vi "solar Delete Target COSMOS Files.vi"(7 "Config Path":path, 8 "error in (no error)":errorcluster, 10 "Target":string, 11 "Refnum in":T1) -> (0 "error out":errorcluster, 3 "Refnum out":T1)   [LabVIEW 2018]
doc: "Deletes a specific targets command and telemetry files."
uses:
  cfg/solar_cfg Read File (Var).vi
  voyager/solar_voy_ctl Voyager Refnum.ctl
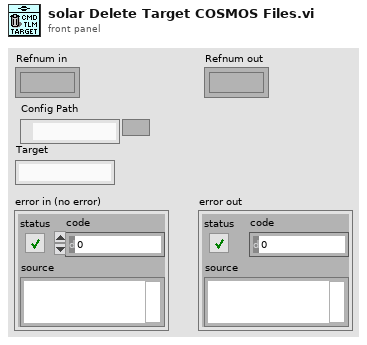
[diagram p1: front panel]
types:
  T1 = typedef "solar_voy_ctl Voyager Refnum.ctl" = refnum<k1>
  T2 = typedef "solar_voy_ctl Voyager.ctl" = cluster{"PACKETS":T3[], "COSMOS_Root":path, "CMD_HDR":T8, "TLM_HDR":T8, "TCPs":T9[], "VoyagerIDOffset":cluster{"VoyagerIDOffset":u16[], "Target Names":string[]}}
  T3 = typedef "solar_voy_def_ctl PACKET.ctl" = cluster{"PACKET_ID":T4, "ENDIAN":enum8{"BIG", "LITTLE"}, "DESC":string, "HZRD":bool, "ITEMS":T5[], "NoExport":bool, "last_time":timestamp, "last_count":u32, "last_data":string}
  T4 = typedef "solar_voy_def_ctl PACKET_ID.ctl" = cluster{"ID":u16, "CMD":enum8{"CMD", "TLM"}, "TARGET":string, "PACKET":string}
  T5 = typedef "solar_voy_def_ctl ITEM.ctl" = cluster{"NAME":string, "OFFSET":i32, "SIZE":i32, "TYPE":T6, "EACH_SIZE":i32, "LVTYPE":T7, "MIN":dbl, "MAX":dbl, "DEFAULT":string, "DESC":string, "ID":bool, "MODIFIERS":variant, "last_value":variant}
  T6 = typedef "solar_voy_def_ctl ITEM TYPE.ctl" = enum8{"BLOCK", "INT", "UINT", "FLOAT", "STRING"}
  T7 = typedef "solar_type Item Type.ctl" = enum16{"NULL", "UNKNOWN", "CLUSTER", "I8", "I16", "I32", "I64", "U8", "U16", "U32", "U64", "U8_ENUM", "U16_ENUM", "U32_ENUM", "SGL", "DBL", "BOOLEAN", "STRING", "PATH", "VISA", "TAG", "TIME", "I8_1D", "I16_1D", "I32_1D", "I64_1D", "U8_1D", "U16_1D", "U32_1D", "U64_1D", "U8_ENUM_1D", "U16_ENUM_1D", "U32_ENUM_1D", "SGL_1D", "DBL_1D", "BOOLEAN_1D", "STRING_1D", "PATH_1D", "VISA_1D", "TAG_1D", "TIME_1D", "I8_2D", "I16_2D", "I32_2D", "I64_2D", "U8_2D", "U16_2D", "U32_2D", "U64_2D", "U8_ENUM_2D", "U16_ENUM_2D", "U32_ENUM_2D", "SGL_2D", "DBL_2D", "BOOLEAN_2D", "STRING_2D", "PATH_2D", "VISA_2D", "TAG_2D", "TIME_2D"}
  T8 = typedef "solar_voy_def_ctl HDR.ctl" = cluster{"ITEMS":T5[], "LENGTH_NAME":string, "LENGTH_VALUE_OFFSET":i32, "ID_NAME":string, "ENDIAN":enum8{"BIG", "LITTLE"}, "GUID_NAME":string, "DEFAULT_TARGET":string, "DEFAULT_PACKET":string, "DEFAULT_ERROR":string}
  T9 = typedef "solar_voy_ctl TCP.ctl" = cluster{"Connected":bool, "Port":u16, "Listener":refnum<k5>, "ServerIP":string, "TCP":refnum<k5>, "Setup":T10, "VIRefnum":refnum<vi>, "TARGETS_CMD":string[], "TARGETS_TLM":string[]}
  T10 = typedef "solar_voy_ctl Port Setup.ctl" = enum8{"SERVER", "CLIENT", "SERVER_CMD", "SERVER_TLM"}
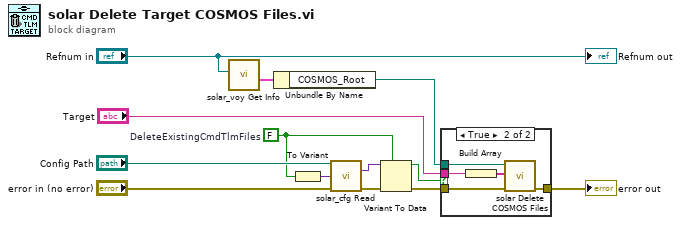
[diagram p0: block diagram]
diagram:
  w4 = FALSE  # DeleteExistingCmdTlmFiles
  n1 = call "solar_voy Get Info.vi"("Voyager Refnum"="Refnum in") -> ("Voyager"=w9:T2)  [unwired: 8 in, 2 out]
  n2 = Unbundle By Name(w9) -> ("COSMOS_Root"=w8:path)
  n3 = To Variant(anything=w4) -> (Variant=w12:variant)
  n4 = call-poly "solar_cfg Read.vi"("Config Path (*.ini)"="Config Path", "Variant in"=w12, "error in (no error)"="error in (no error)") -> ("Variant out"=w5:variant, "error out"=w10:errorcluster)  [unwired: 9 in, 2 out]
  n5 = Variant To Data(error in=w10, type=w4, Variant=w5) -> (data=w3:bool, error out=w6:errorcluster)
  n6 = case shown="True" w3 {
    tunnel: [w14 w19] -> w11
    tunnel: w8 -> [_ w18]
    tunnel: w6 -> [w14 w17]
    tunnel: "Target" -> [_ w15]
    frame False {
    }
    frame True {
      n7 = Build Array(w15) -> (w16:string[])
      n8 = call "solar Delete COSMOS Files.vi"("error in (no error)"=w17, "Target Folders to Delete"=w16, "COSMOS_Root"=w18) -> ("error out"=w19:errorcluster)  [unwired: 8 in]
    }
  }
  "error out" <- w11
  "Refnum out" <- "Refnum in"
